vi "Untitled 6.vi"(1 "data":dynamicdata(waveform), 2 "rate":dbl=1000.0, 4 "timeout (s)":dbl=10.0 format="%0.2f", 5 "error in":errorcluster, 7 "stop (T)":bool=TRUE, 10 "device name":tag="Dev1") -> (14 "task out":refnum<k21>, 19 "error out":errorcluster)   [LabVIEW 2017]
doc: "Creates, edits, and runs tasks using NI-DAQmx. Refer to the NI-DAQmx Readme for a complete listing of devices NI-DAQmx supports.\n\nWhen you place this Express VI on the block diagram, the DAQ Assistant launches to create a new task. After you create a task, you can double-click the DAQ Assistant Express VI to edit that task. For continuous measurement or generation, place a while loop around the DAQ Assistant Express VI."
uses:
  <vilib>/DAQmx/write.llb/DAQmx Write.vi
  <vilib>/DAQmx/write.llb/DAQmx Write (Analog 1D Wfm NChan NSamp).vi
  <vilib>/DAQmx/miscellaneous.llb/DAQmx Fill In Error Info.vi
  <vilib>/DAQmx/configure/trigger.llb/DAQmx Trigger.vi
  <vilib>/DAQmx/configure/trigger.llb/DAQmx Start Trigger (Digital Edge).vi
  <vilib>/DAQmx/configure/timing.llb/DAQmx Timing (Sample Clock).vi
  <vilib>/DAQmx/create/channels.llb/DAQmx Create Channel (AO-Voltage-Basic).vi
  <resource>/objmgr/daqmx.rc
panel:
  in  "Analog Trigger Source":tag="/Dev1/ao/SampleClock"
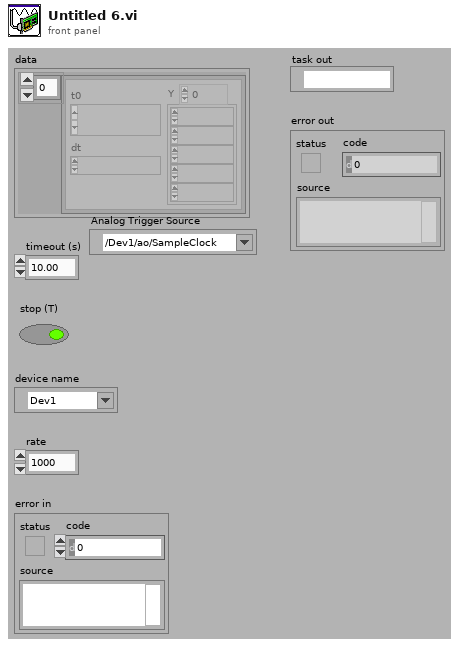
[diagram p1: front panel]
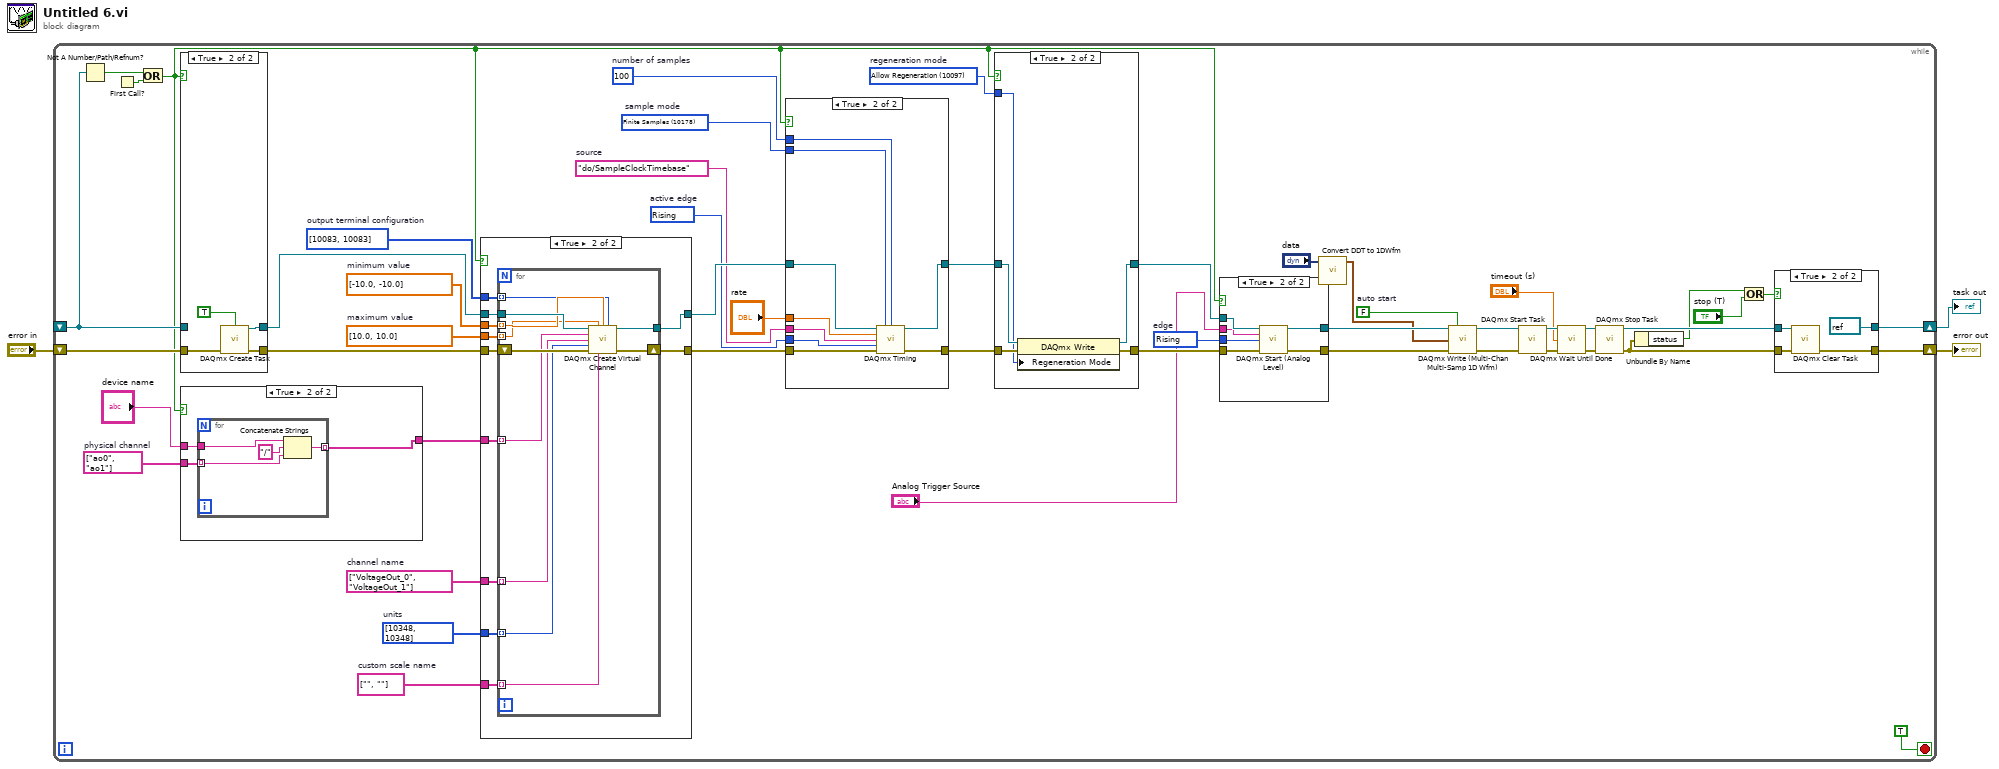
[diagram p0: block diagram]
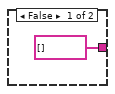
[diagram p7: hidden frame]
diagram:
  n1 = while {
    shift-right: [w11] -> w1
    shift-left: _ -> [w50]
    shift-right: [w5] -> w2
    shift-left: "error in" -> [w51]
    stop <- TRUE stop-if-true
    w21 = FALSE  # auto start
    w24 = 10280 items=["Rising"=10280, "Falling"=10171]  # edge
    w28 = 10097 items=["Allow Regeneration"=10097, "Do Not Allow Regeneration"=10158]  # regeneration mode
    w31 = 10178 items=["Finite Samples"=10178, "Continuous Samples"=10123, "Hardware Timed Single Point"=12522]  # sample mode
    w32 = 10280 items=["Rising"=10280, "Falling"=10171]  # active edge
    w33 = "do/SampleClockTimebase"  # source
    w35 = 100  # number of samples
    w38 = i32[] [10083, 10083] items=["Default"=-1, "RSE"=10083, "Differential"=10106, "Pseudodifferential"=12529]  # output terminal configuration
    w39 = string[] ["", ""]  # custom scale name
    w40 = i32[] [10348, 10348] items=["Volts"=10348, "From Custom Scale"=10065]  # units
    w41 = string[] ["VoltageOut_0", "VoltageOut_1"]  # channel name
    w43 = dbl[] [10.0, 10.0]  # maximum value
    w44 = dbl[] [-10.0, -10.0]  # minimum value
    w47 = string[] ["ao0", "ao1"]  # physical channel
    n2 = Not A Number/Path/Refnum?(number/path/refnum=w50) -> (NaN/Path/Refnum?=w49:bool)
    n3 = First Call?() -> (First Call?: T/F=w52:bool)
    n4 = Or(x=w49, y=w52) -> (x .or. y?=w27:bool)
    n5 = case shown="True" w27 {
      tunnel: [w119 w123] -> w46
      tunnel: w50 -> [w119 _]
      tunnel: [w118 w122] -> w45
      tunnel: w51 -> [w118 w120]
      frame False {
      }
      frame True {
        n6 = call <vilib>:"DAQmx Create Task.vi"("auto cleanup"=TRUE, "error in"=w120) -> ("task out"=w123:refnum<k21>, "error out"=w122:errorcluster)  [unwired: 12 in]
      }
    }
    n7 = case shown="True" w27 {
      tunnel: [string[] [] w113] -> w42
      tunnel: "device name" -> [_ w112]
      tunnel: w47 -> [_ w111]
      frame False {
      }
      frame True {
        n8 = for {
          tunnel: [w117] -> w113 mode=indexing
          tunnel: w112 -> [w116]
          tunnel: w111 -> [w114] mode=indexing
          n9 = Concatenate Strings(w116, "/" ("string"), w114) -> (w117:string)
        }
      }
    }
    n10 = case shown="True" w27 {
      tunnel: [w87 w96] -> w37
      tunnel: w46 -> [w87 w98]
      tunnel: [w86 w95] -> w36
      tunnel: w45 -> [w86 w97]
      tunnel: w44 -> [_ w94]
      tunnel: w43 -> [_ w93]
      tunnel: w42 -> [_ w92]
      tunnel: w41 -> [_ w91]
      tunnel: w40 -> [_ w90]
      tunnel: w39 -> [_ w89]
      tunnel: w38 -> [_ w88]
      frame False {
      }
      frame True {
        n11 = for {
          tunnel: w98 -> [w109]
          tunnel: [w107] -> w96
          tunnel: w94 -> [w105] mode=indexing
          tunnel: w93 -> [w104] mode=indexing
          tunnel: w92 -> [w103] mode=indexing
          tunnel: w91 -> [w102] mode=indexing
          tunnel: w90 -> [w101] mode=indexing
          tunnel: w89 -> [w100] mode=indexing
          shift-right: [w106] -> w95
          shift-left: w97 -> [w108]
          tunnel: w88 -> [w99] mode=indexing
          n12 = call-poly <vilib>:"DAQmx Create Virtual Channel.vi"("task in"=w109, "maximum value"=w104, "minimum value"=w105, "output terminal configuration"=w99, "physical channels"=w103, "name to assign"=w102, "units"=w101, "error in"=w108, "custom scale name"=w100) -> ("task out"=w107:refnum<k21>, "error out"=w106:errorcluster)  [unwired: 5 in]
        }
      }
    }
    n13 = case shown="True" w27 {
      tunnel: [w76 w83] -> w30
      tunnel: w37 -> [w76 w85]
      tunnel: [w75 w82] -> w29
      tunnel: w36 -> [w75 w84]
      tunnel: w31 -> [_ w81]
      tunnel: w35 -> [_ w80]
      tunnel: "rate" -> [_ w79]
      tunnel: w33 -> [_ w78]
      tunnel: w32 -> [_ w77]
      frame False {
      }
      frame True {
        n14 = call-poly <vilib>:"DAQmx Timing.vi"("task/channels in"=w85, "sample mode"=w81, "samples per channel"=w80, "rate"=w79, "source"=w78, "active edge"=w77, "error in"=w84) -> ("task out"=w83:refnum<k21>, "error out"=w82:errorcluster)  [unwired: 7 in]
      }
    }
    n15 = case shown="True" w27 {
      tunnel: w30 -> [w69 w74]
      tunnel: [w69 w73] -> w26
      tunnel: w29 -> [w68 w72]
      tunnel: [w68 w71] -> w25
      tunnel: w28 -> [_ w70]
      frame False {
      }
      frame True {
        n16 = property class="DAQmx Write"(reference=w74, error in=w72, "Regeneration Mode"=w70) -> (reference out=w73:refnum<k21>, error out=w71:errorcluster)
      }
    }
    n17 = case shown="True" w27 {
      tunnel: [w61 w65] -> w23
      tunnel: w26 -> [w61 w67]
      tunnel: [w60 w64] -> w22
      tunnel: w25 -> [w60 w66]
      tunnel: "Analog Trigger Source" -> [_ w63]
      tunnel: w24 -> [_ w62]
      frame False {
      }
      frame True {
        n18 = call-poly "DAQmx Start (Analog Level).vi"("task/channels in"=w67, "source"=w63, "edge"=w62, "error in"=w66) -> ("task out"=w65:refnum<k21>, "error out"=w64:errorcluster)  [unwired: 10 in]
      }
    }
    n19 = call <vilib>:"Convert DDT to 1DWfm.vi"("Dynamic Data Type"="data") -> ("Array of Waveforms"=w19:waveform(dbl)[])  [unwired: 3 in]
    n20 = call-poly "DAQmx Write (Multi-Chan Multi-Samp 1D Wfm).vi"("task/channels in"=w23, "auto start"=w21, "data"=w19, "error in"=w22) -> ("task out"=w14:refnum<k21>, "error out"=w13:errorcluster)  [unwired: 9 in, 1 out]
    n21 = call <vilib>:"DAQmx Start Task.vi"("task/channels in"=w14, "error in"=w13) -> ("task out"=w18:refnum<k21>, "error out"=w17:errorcluster)  [unwired: 12 in]
    n22 = call <vilib>:"DAQmx Wait Until Done.vi"("task/channels in"=w18, "timeout (sec)"="timeout (s)", "error in"=w17) -> ("task out"=w15:refnum<k21>, "error out"=w16:errorcluster)  [unwired: 11 in]
    n23 = call <vilib>:"DAQmx Stop Task.vi"("task/channels in"=w15, "error in"=w16) -> ("task out"=w12:refnum<k21>, "error out"=w9:errorcluster)  [unwired: 12 in]
    n24 = Unbundle By Name(w9) -> ("status"=w8:bool)
    n25 = Or(x=w8, y="stop (T)") -> (x .or. y?=w6:bool)
    n26 = case shown="True" w6 {
      tunnel: w12 -> [w55 w59]
      tunnel: [w55 refnum<k21> refnum ("task in")] -> w11
      tunnel: w9 -> [w54 w58]
      tunnel: [w54 w57] -> w5
      frame False {
      }
      frame True {
        n27 = call <vilib>:"DAQmx Clear Task.vi"("task in"=w59, "error in"=w58) -> ("error out"=w57:errorcluster)  [unwired: 13 in]
      }
    }
  }
  "error out" <- w2
  "task out" <- w1
